vi "Act.vi"(0 "Enum":enum16{"Running", "Impact", "Spinning", "Clear"}(ring)) -> ()   [LabVIEW 2010]
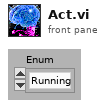
[diagram p1: front panel]
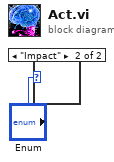
[diagram p0: block diagram]
diagram:
  n1 = case shown="\"Impact\"" "Enum" {
    frame "Running", Default {
    }
    frame "Impact" {
    }
  }
